vi "New.vi"(8 "error in (no error)":errorcluster, 11 "reference in":refnum<class "JTAG_Cyclone.lvclass">) -> (0 "error out":errorcluster, 3 "reference out":refnum<class "JTAG_Cyclone.lvclass">)   [LabVIEW 2022 SP3, in "JTAG_Cyclone.lvlib" / "JTAG_Cyclone.lvclass"]
uses:
  JTAG_Cyclone.lvclass
  ObjectAttributes.ctl
  Config.ctl
  JTAG_Cyclone.lvclass/JTAG_Cyclone.ctl
  Components/JTAG_Base.lvlibp/JTAG_Base.lvclass
panel:
  in  "Data":T1
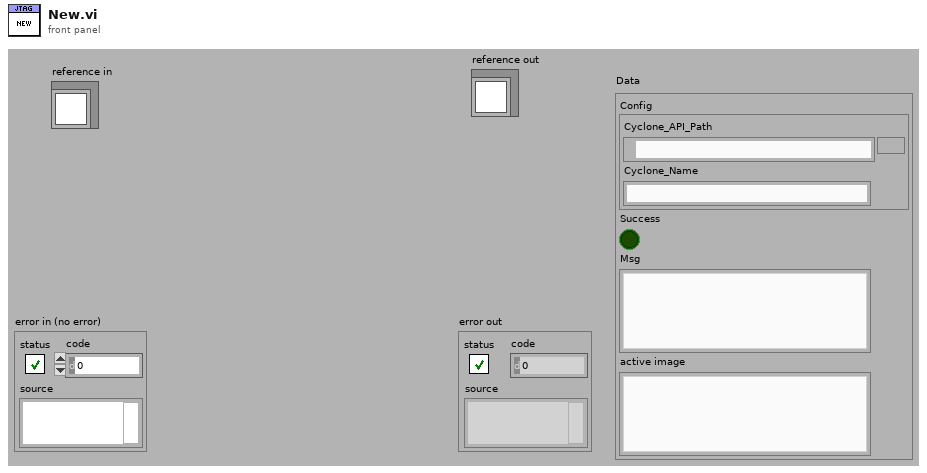
[diagram p1: front panel]
types:
  T1 = typedef "JTAG_Cyclone.lvlib/JTAG_Cyclone.lvclass/ObjectAttributes.ctl" = cluster{"Config":T2, "Success":bool, "Msg":string, "active image":string}
  T2 = typedef "JTAG_Cyclone.lvlib/JTAG_Cyclone.lvclass/Config.ctl" = cluster{"Cyclone_API_Path":path, "Cyclone_Name":string}
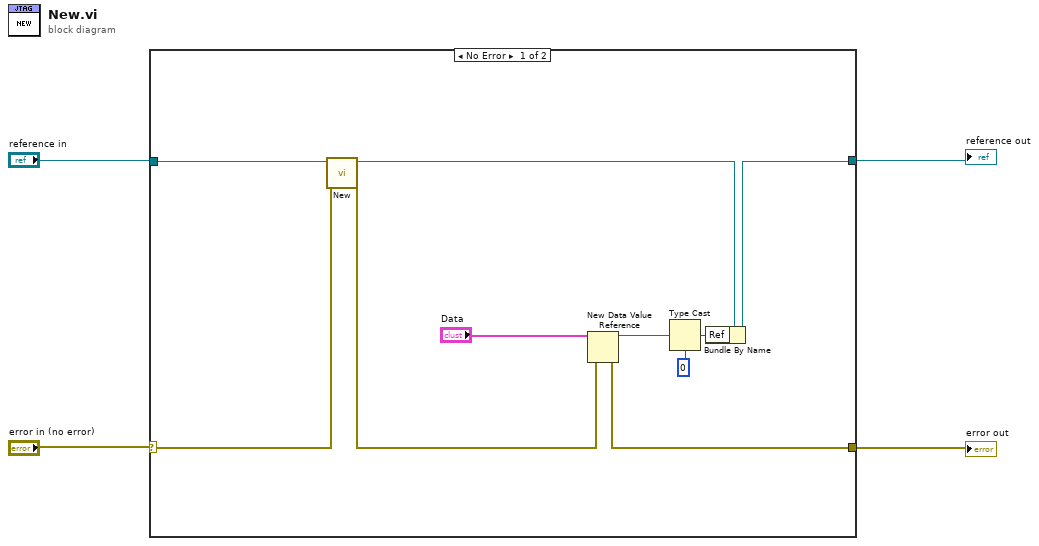
[diagram p0: block diagram]
diagram:
  n1 = case shown="No Error" "error in (no error)" {
    selector: "error in (no error)" -> [w6 w16]
    tunnel: [w7 w16] -> w2
    tunnel: "reference in" -> [w14 w15]
    tunnel: [w13 w15] -> w1
    frame No Error {
      n2 = call-parent "New.vi"("error in (no error)"=w6, "reference in"=w14) -> ("error out"=w5:errorcluster, "reference out"=w12:refnum<class "JTAG_Cyclone.lvclass">)  [unwired: 8 in]
      n3 = New Data Value Reference(data value="Data", error in=w5) -> (data value reference=w10:refnum<data-value>, error out=w7:errorcluster)
      n4 = Type Cast(type=u32 0 ("DataRef"), x=w10) -> (*(type *) &x=w9:u32)
      n5 = Bundle By Name(cluster=w12, "Ref"=w9) -> (w13:refnum<class "JTAG_Cyclone.lvclass">)
    }
    frame Error {
    }
  }
  "error out" <- w2
  "reference out" <- w1
